vi "Configure Corrections.vi"(0 "VISA resource name":refnum<visa-resource-name>, 1 "Channel (1)":i32=1, 5 "Electrical DelayTime (0.0)":dbl format="%^.2e", 7 "Velocity Factor (1.0)":dbl=1.0 format="%^.2e", 9 "Phase Offset (0.0)":dbl format="%^.2e", 11 "error in (no error)":errorcluster) -> (4 "VISA resource name out":refnum<visa-resource-name>, 15 "error out":errorcluster)   [LabVIEW 2012, in "Tektronix TTR500 Series.lvlib"]
doc: "This VI configures display corrections."
uses:
  <instrlib>/Tektronix TTR500 Series/Tektronix TTR500 Series.lvlib
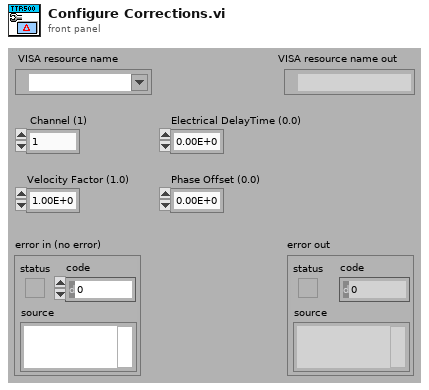
[diagram p1: front panel]
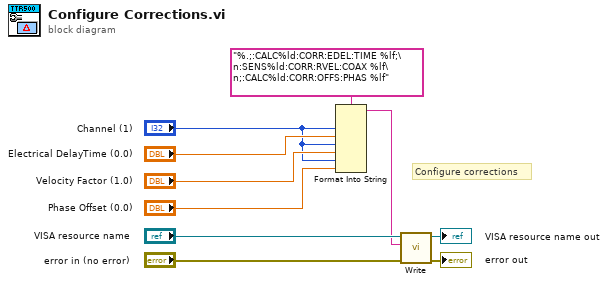
[diagram p0: block diagram]
diagram:
  # "Configure corrections"
  n1 = Format Into String(format string="%.;:CALC%ld:CORR:EDEL:TIME %lf;\n:SENS%ld:CORR:RVEL:COAX %lf\n;:CALC%ld:CORR:OFFS:PHAS %lf", "Channel (1)", "Electrical DelayTime (0.0)", "Channel (1)", "Velocity Factor (1.0)", "Channel (1)", "Phase Offset (0.0)") -> (resulting string=w5:string)  [unwired: 2 in, 1 out]
  n2 = call <instrlib>:"Write.vi"("error in (no error)"="error in (no error)", "String ()"=w5, "VISA resource name"="VISA resource name") -> ("error out"=→"error out":errorcluster, "VISA resource name out"=→"VISA resource name out":refnum<visa-resource-name>)  [unwired: 6 in, 1 out]
